vi "Configure Parallel.vi"(8 "error in (no error)":errorcluster, 9 "Parallel Channels (0:CH1+CH2)":u16(ring) items=["CH1+CH2", "CH2+CH3", "ALL"], 10 "Enable Parallel Mode (T: Enable)":bool=TRUE, 11 "VISA resource name":refnum<visa-resource-name>) -> (0 "error out":errorcluster, 3 "VISA resource name out":refnum<visa-resource-name>)   [LabVIEW 2017, in "BK Precision 913XX.lvlib"]
doc: "Enables or disables parallel mode for the selected channels.\n\n<B>Note: To enable parallel mode, tracking or series mode must first be disabled using Configure Tracking.vi or Configure Series.vi respectively. Otherwise, an error will occur.</B>"
uses:
  <instrlib>/BK Precision 913XX/BK Precision 913XX.lvlib
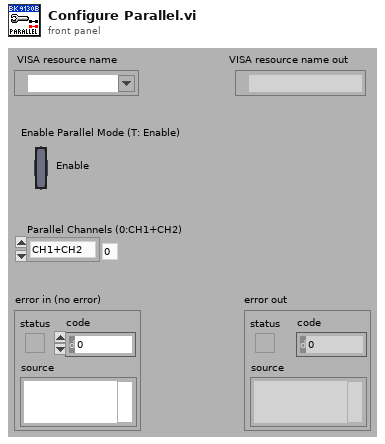
[diagram p1: front panel]
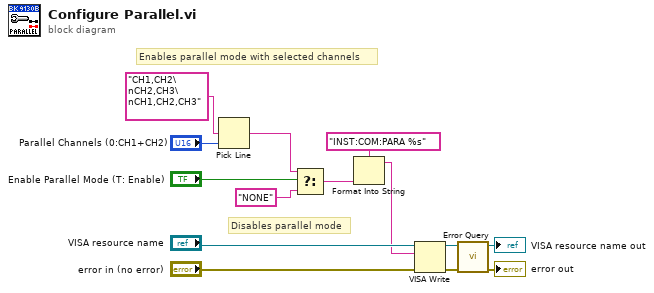
[diagram p0: block diagram]
diagram:
  # "Enables parallel mode with selected channels"
  # "Disables parallel mode"
  n1 = Pick Line(multi-line string="CH1,CH2\nCH2,CH3\nCH1,CH2,CH3", line index="Parallel Channels (0:CH1+CH2)") -> (output string=w2:string)  [unwired: 1 in]
  n2 = Select(t=w2, s="Enable Parallel Mode (T: Enable)", f="NONE") -> (s? t:f=w7:string)
  n3 = Format Into String(format string="INST:COM:PARA %s", w7) -> (resulting string=w1:string)  [unwired: 2 in, 1 out]
  n4 = VISA Write(VISA resource name="VISA resource name", write buffer=w1, error in (no error)="error in (no error)") -> (VISA resource name out=w12:refnum<visa-resource-name>, error out=w11:errorcluster)  [unwired: 1 out]
  n5 = call <instrlib>:"Error Query.vi"("error in (no error)"=w11, "VISA resource name"=w12) -> ("error out"=→"error out":errorcluster, "VISA resource name out"=→"VISA resource name out":refnum<visa-resource-name>)  [unwired: 6 in, 2 out]
